vi "Write File Header.vi"(0 "Æ Trigger":dbl format="%.2f", 1 "Trigger Column":i32, 2 "Comments":string="This data's for you!\nType \u0011-H to get a help window for the various controls.", 4 "Scale Factors":dbl[](array[numeric]) format="%.2f", 5 "Output File Name":string, 6 "Magnet Id":string, 7 "# Cols":i32, 8 "User Name":string="Conan The Scientist", 9 "File Ref Num 2":refnum<file>) -> (3 "File Ref Num":refnum<file>)   [LabVIEW 2021]
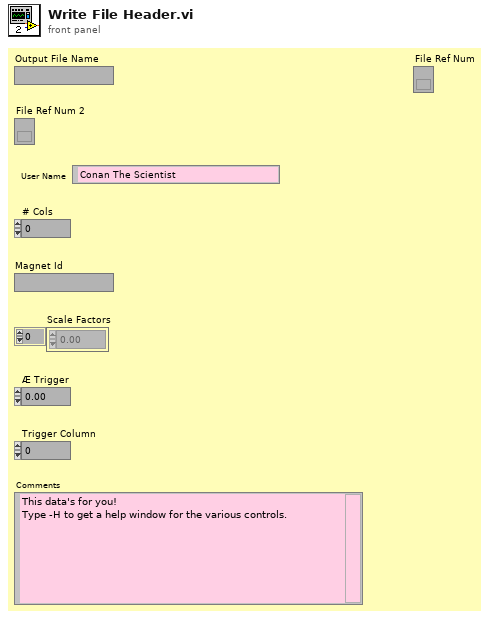
[diagram p1: front panel]
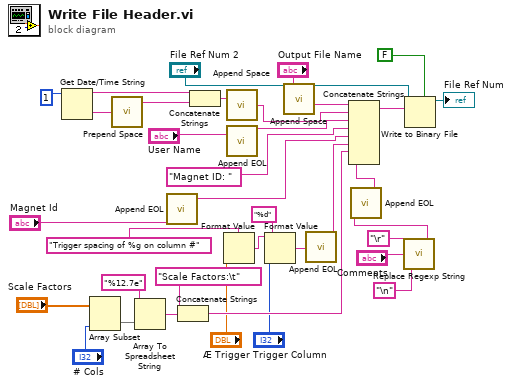
[diagram p0: block diagram]
diagram:
  n1 = Get Date/Time String(date format (0)=1) -> (date string=w11:string, time string=w13:string)  [unwired: 2 in]
  n2 = Array Subset(array="Scale Factors", length="# Cols") -> (w29:dbl[])  [unwired: 1 in]
  n3 = call "Prepend Space.vi"("Input String"=w13) -> ("Space + Input String"=w12:string)
  n4 = Array To Spreadsheet String(array=w29, 3:"%12.7e") -> (spreadsheet string=w25:string)  [unwired: 1 in]
  n5 = call "Append EOL.vi"("INPUT STRING"="Magnet Id") -> ("OUTPUT STRING (PLUS End of Line)"=w9:string)
  n6 = Concatenate Strings("Scale Factors:\t", w25) -> (w27:string)
  n7 = Concatenate Strings(w11, w12) -> (w10:string)
  n8 = Format Value(format string="Trigger spacing of %g on column #", value (0)="Æ Trigger") -> (output string=w18:string)  [unwired: 1 in]
  n9 = call "Append Space.vi"("INPUT STRING"=w10) -> ("OUTPUT STRING (PLUS [SPACE])"=w6:string)
  n10 = call "Append EOL.vi"("INPUT STRING"="User Name") -> ("OUTPUT STRING (PLUS End of Line)"=w7:string)
  n11 = Format Value(string ("")=w18, format string="%d", value (0)="Trigger Column") -> (output string=w19:string)
  n12 = call "Append Space.vi"("INPUT STRING"="Output File Name") -> ("OUTPUT STRING (PLUS [SPACE])"=w5:string)
  n13 = call "Append EOL.vi"("INPUT STRING"=w19) -> ("OUTPUT STRING (PLUS End of Line)"=w22:string)
  n14 = call "Replace Regexp String.vi"("Search String"="\n", "Input String"="Comments", "Replacement String"="\r") -> ("Output String"=w32:string)
  n15 = call "Append EOL.vi"("INPUT STRING"=w32) -> ("OUTPUT STRING (PLUS End of Line)"=w28:string)
  n16 = Concatenate Strings(w5, w6, w7, "Magnet ID: ", w9, w22, w27, w28) -> (w2:string)
  n17 = Write to Binary File(file (use dialog)="File Ref Num 2", data=w2, 5:FALSE ("prepend array or string size? (T)")) -> (refnum out=→"File Ref Num":refnum<file>)  [unwired: 3 in, 2 out]
